vi "VerifyMenuItems.vi"(8 "error in (no error)":errorcluster, 10 "Menu Item In":string, 11 "MenuCol in":refnum<class "MenuCol.lvclass">) -> (0 "error out":errorcluster, 1 "Valid Menu Item":bool, 2 "Menu Item Out":string, 3 "MenuCol out":refnum<class "MenuCol.lvclass">)   [LabVIEW 2013, in "MenuCol.lvclass"]
uses:
  MenuCol.lvclass
  MenuCol.lvclass/MenuCol.ctl
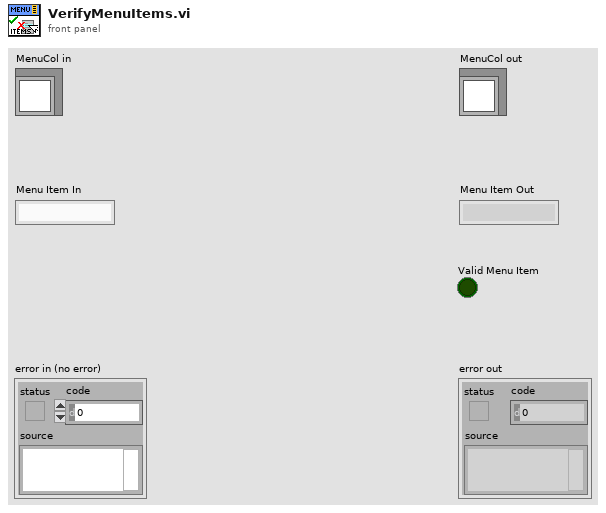
[diagram p1: front panel]
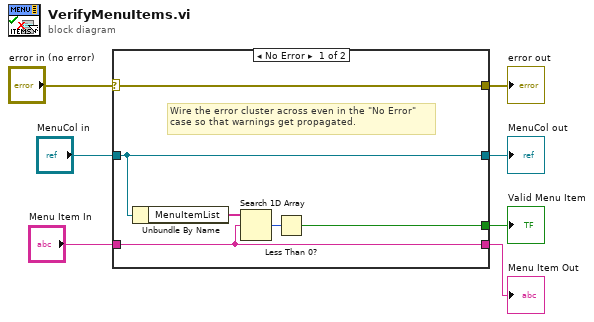
[diagram p0: block diagram]
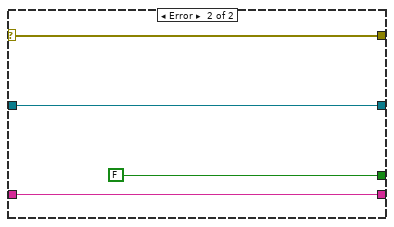
[diagram p2: hidden frame]
diagram:
  n1 = case shown="No Error" "error in (no error)" {
    selector: "error in (no error)" -> [w13 w17]
    tunnel: [w13 w17] -> w6
    tunnel: [w12 w16] -> w4
    tunnel: "MenuCol in" -> [w12 w16]
    tunnel: [w8 FALSE] -> w3
    tunnel: "Menu Item In" -> [w10 w14]
    tunnel: [w10 w14] -> w1
    frame No Error {
      # "Wire the error cluster across even in the \"No Error\"\ncase so that warnings get propagated."
      n2 = Unbundle By Name(w12) -> ("MenuItemList"=w11:string[])
      n3 = Search 1D Array(1D array=w11, element=w10) -> (index of element=w9:i32)  [unwired: 1 in]
      n4 = Less Than 0?(x=w9) -> (x < 0?=w8:bool)
    }
    frame Error {
    }
  }
  "error out" <- w6
  "MenuCol out" <- w4
  "Valid Menu Item" <- w3
  "Menu Item Out" <- w1
